vi "CreatePublicEvents.vi"(8 "error in (no error)":errorcluster, 11 "RemoteControl":refnum<class "RemoteControl.lvclass">) -> (0 "error out":errorcluster, 3 "RemoteControl out":refnum<class "RemoteControl.lvclass">)   [LabVIEW 2016, in "RemoteControl.lvclass"]
doc: "---------------------------------------------------------------\nJKI State Machine Objects™\nhttp://jki.net/state-machine-objects/\nCopyright (C) 2005-2015, JKI <info@jki.net>\nALL RIGHTS RESERVEDJKI State Machine Objects (SMO) 1.0.0.4\nJKI - JKI\nCopyright (c) 2015, JKI"
uses:
  RemoteControl.lvclass
  Typedefs/PublicEvents--RemoteControl.configRemote.ctl
  Typedefs/PublicEvents--RemoteControl.configIVmode.ctl
  Typedefs/PublicEvents--RemoteControl.configREF.ctl
  Typedefs/REF-cluster.ctl
  Typedefs/REF_f-array.ctl
  Typedefs/REF_phi-array.ctl
  Typedefs/PublicEvents--RemoteControl.configAO.ctl
  Typedefs/AO-cluster.ctl
  Typedefs/AO_Amp-array.ctl
  Typedefs/AO_DC-array.ctl
  Typedefs/AO_f-array.ctl
  Typedefs/AO_phi-array.ctl
  Typedefs/Function-array.ctl
  Typedefs/Function-enum.ctl
  Typedefs/PublicEvents--RemoteControl.assertTrigger.ctl
  Typedefs/PublicEvents--RemoteControl.configReset.ctl
  RemoteControl.lvclass/RemoteControl.ctl
  <vilib>/JKI/JKI SMO/SMO/SMO.lvclass
panel:
  # "For instructions on how to use the JKI State Machine Objects, examples and video tutorials, visit:\nhttp://jki.net/state-machine-objects/\n\nJKI State Machine Objects™\nhttp://jki.net/state-machine-objects/\nCopyright (C) 2005-2015, JKI <info@jki.net>\nALL RIGHTS RESERVED"
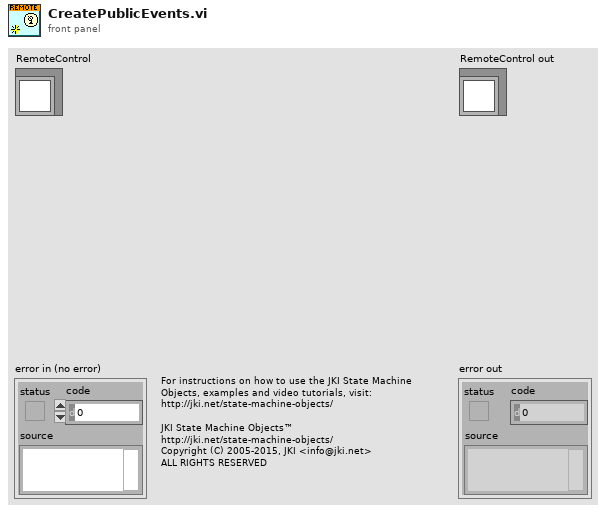
[diagram p1: front panel]
types:
  T1 = typedef "RemoteControl.lvclass/PublicEvents--RemoteControl.configReset.ctl" = bool
  T2 = typedef "RemoteControl.lvclass/PublicEvents--RemoteControl.assertTrigger.ctl" = bool
  T3 = typedef "RemoteControl.lvclass/PublicEvents--RemoteControl.configAO.ctl" = cluster{"Channels: AO":T4}
  T4 = typedef "AO-cluster.ctl" = cluster{"AO amp (V)":T5, "AO DC (V)":T6, "AO f (Hz)":T7, "AO phi (deg)":T8, "function":T9}
  T5 = typedef "AO_Amp-array.ctl" = dbl[]
  T6 = typedef "AO_DC-array.ctl" = dbl[]
  T7 = typedef "AO_f-array.ctl" = dbl[]
  T8 = typedef "AO_phi-array.ctl" = dbl[]
  T9 = typedef "Function-array.ctl" = T10[]
  T10 = typedef "Function-enum.ctl" = enum16{"Sine Wave", "Triangle Wave", "Square Wave", "Sawtooth Wave"}
  T11 = typedef "RemoteControl.lvclass/PublicEvents--RemoteControl.configREF.ctl" = cluster{"Channels: Lockin":T12}
  T12 = typedef "REF-cluster.ctl" = cluster{"REF f (Hz)":T13, "REF phi (deg)":T14}
  T13 = typedef "REF_f-array.ctl" = dbl[]
  T14 = typedef "REF_phi-array.ctl" = dbl[]
  T15 = typedef "RemoteControl.lvclass/PublicEvents--RemoteControl.configIVmode.ctl" = bool
  T16 = typedef "RemoteControl.lvclass/PublicEvents--RemoteControl.configRemote.ctl" = bool
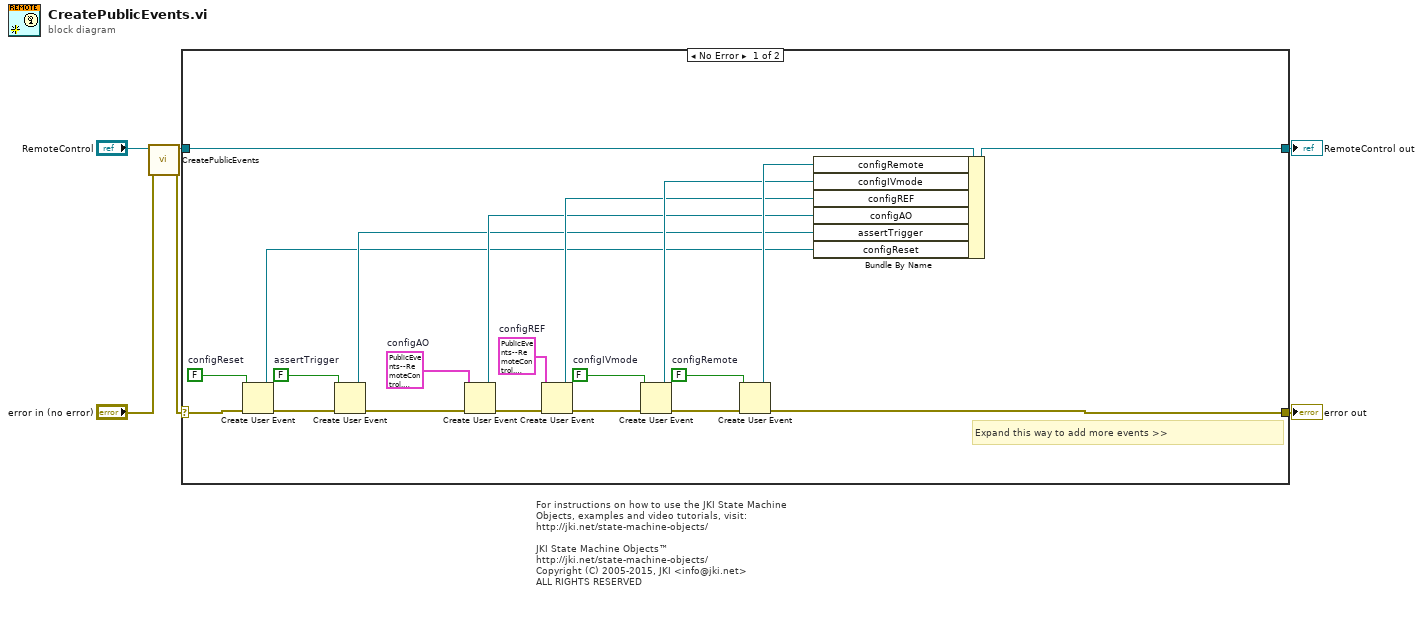
[diagram p0: block diagram]
diagram:
  # "For instructions on how to use the JKI State Machine Objects, examples and video tutorials, visit:\nhttp://jki.net/state-machine-objects/\n\nJKI State Machine Objects™\nhttp://jki.net/state-machine-objects/\nCopyright (C) 2005-2015, JKI <info@jki.net>\nALL RIGHTS RESERVED"
  n1 = call-parent "CreatePublicEvents.vi"("error in (no error)"="error in (no error)", "SMO"="RemoteControl") -> ("error out"=w1:errorcluster, "SMO out"=w3:refnum<class "RemoteControl.lvclass">)  [unwired: 8 in]
  n2 = case shown="No Error" w1 {
    selector: w1 -> [w26 w29]
    tunnel: [w24 w29] -> w5
    tunnel: [w25 w28] -> w6
    tunnel: w3 -> [w27 w28]
    frame No Error {
      w8 = T1 FALSE  # configReset
      w11 = T2 FALSE  # assertTrigger
      w14 = T3 {"Channels: AO"={"AO amp (V)"=[0.01, 0.0, 0.0, 0.0, 0.0, 0.0, 0.0, 0.0], "AO DC (V)"=[0.0, 0.0, 0.0, 0.0, 0.0, 0.0, 0.0, 0.0], "AO f (Hz)"=[13.1, 13.0, 13.0, 13.0, 13.0, 13.0, 13.0, 13.0], "AO phi (deg)"=[0.0, 0.0, 0.0, 0.0, 0.0, 0.0, 0.0, 0.0], "function"=[enum."Sine Wave", enum."Sine Wave", enum."Sine Wave", enum."Sine Wave", enum."Sine Wave", enum."Sine Wave", enum."Sine Wave", enum."Sine Wave"]}}  # configAO
      w17 = T11 {"Channels: Lockin"={"REF f (Hz)"=[13.0], "REF phi (deg)"=[0.0, 0.0, 0.0, 0.0, 0.0, 0.0, 0.0, 0.0]}}  # configREF
      w20 = T15 FALSE  # configIVmode
      w23 = T16 FALSE  # configRemote
      # "Expand this way to add more events >>"
      n3 = Create User Event(user event datatype=w8, error in=w26) -> (user event=w7:refnum<user-event>, error out=w9:errorcluster)
      n4 = Create User Event(user event datatype=w11, error in=w9) -> (user event=w10:refnum<user-event>, error out=w12:errorcluster)
      n5 = Create User Event(user event datatype=w14, error in=w12) -> (user event=w13:refnum<user-event>, error out=w15:errorcluster)
      n6 = Create User Event(user event datatype=w17, error in=w15) -> (user event=w16:refnum<user-event>, error out=w18:errorcluster)
      n7 = Create User Event(user event datatype=w20, error in=w18) -> (user event=w19:refnum<user-event>, error out=w21:errorcluster)
      n8 = Create User Event(user event datatype=w23, error in=w21) -> (user event=w22:refnum<user-event>, error out=w24:errorcluster)
      n9 = Bundle By Name(cluster=w27, "configRemote"=w22, "configIVmode"=w19, "configREF"=w16, "configAO"=w13, "assertTrigger"=w10, "configReset"=w7) -> (w25:refnum<class "RemoteControl.lvclass">)
    }
    frame Error {
    }
  }
  "error out" <- w5
  "RemoteControl out" <- w6
